vi "Interpolate 2D Scattered_Wn2.vi"(0 "X(Tri) In":dbl[][](array[numeric]), 5 "Y(Tri) In":dbl[][](array[numeric]), 7 "Z(Tri) In":dbl[][](array[numeric]), 9 "gx in":dbl[][](array[numeric]), 11 "gy in":dbl[][](array[numeric]), 12 "Length":dbl[][](array[numeric])) -> (4 "X(Tri) Out":dbl[][](array[numeric]), 6 "Y(Tri) Out":dbl[][](array[numeric]), 8 "Z(Tri) Out":dbl[][](array[numeric]), 10 "gx out":dbl[][](array[numeric]), 14 "Wn 2":dbl[][](array[numeric]), 15 "gy out":dbl[][](array[numeric]))   [LabVIEW 2017, in "NI_AAL_Interpolation.lvlib"]
uses:
  <vilib>/gmath/NI_AAL_Interpolation.lvlib
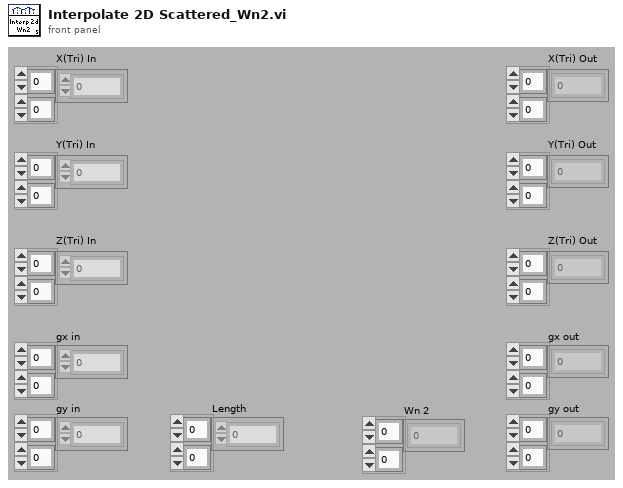
[diagram p1: front panel]
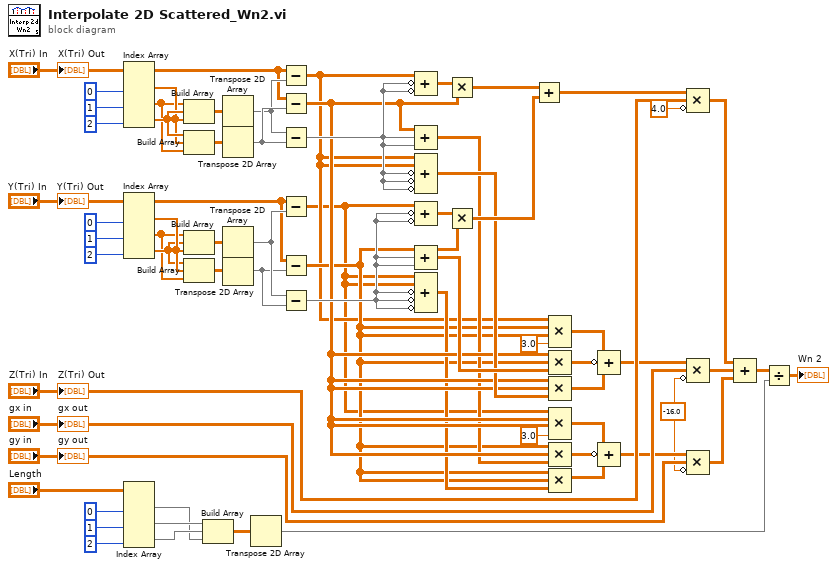
[diagram p0: block diagram]
diagram:
  w8 = -16.0
  n1 = Index Array(array="X(Tri) In", index (col) #1=0 ("disabled index (col)"), index (col) #2=1 ("index (col)"), index (col) #3=2 ("index (col)")) -> (element #1=w59:dbl[], element #2=w58:dbl[], element #3=w60:dbl[])  [unwired: 3 in]
  n2 = Index Array(array="Y(Tri) In", index (col) #1=0 ("disabled index (col)"), index (col) #2=1 ("index (col)"), index (col) #3=2 ("index (col)")) -> (element #1=w57:dbl[], element #2=w55:dbl[], element #3=w56:dbl[])  [unwired: 3 in]
  n3 = Index Array(array="Length", index (col) #1=0 ("disabled index (col)"), index (col) #2=1 ("index (col)"), index (col) #3=2 ("index (col)")) -> (element #1=w40:dbl[], element #2=w42:dbl[], element #3=w41:dbl[])  [unwired: 3 in]
  n4 = Build Array(w58, w60, w59) -> (w52:dbl[][])
  n5 = Build Array(w60, w59, w58) -> (w51:dbl[][])
  n6 = Build Array(w55, w56, w57) -> (w54:dbl[][])
  n7 = Build Array(w56, w57, w55) -> (w53:dbl[][])
  n8 = Build Array(w42, w41, w40) -> (w43:dbl[][])
  n9 = Transpose 2D Array(2D array=w52) -> (transposed array=w44:dbl[][])
  n10 = Transpose 2D Array(2D array=w51) -> (transposed array=w45:dbl[][])
  n11 = Transpose 2D Array(2D array=w54) -> (transposed array=w47:dbl[][])
  n12 = Transpose 2D Array(2D array=w53) -> (transposed array=w46:dbl[][])
  n13 = Transpose 2D Array(2D array=w43) -> (transposed array=w33:dbl[][])
  n14 = Subtract(x="X(Tri) In", y=w44) -> (x-y=w3:dbl[][])
  n15 = Subtract(x="X(Tri) In", y=w45) -> (x-y=w22:dbl[][])
  n16 = Subtract(x=w44, y=w45) -> (x-y=w28:dbl[][])
  n17 = Subtract(x="Y(Tri) In", y=w47) -> (x-y=w2:dbl[][])
  n18 = Subtract(x="Y(Tri) In", y=w46) -> (x-y=w19:dbl[][])
  n19 = Subtract(x=w47, y=w46) -> (x-y=w26:dbl[][])
  n20 = Compound Arithmetic op=ADD(w3, invert w28, invert w28) -> (w32:dbl[][])
  n21 = Compound Arithmetic op=ADD(w22, w28, w28) -> (w21:dbl[][])
  n22 = Compound Arithmetic op=ADD(w3, w3, invert w28, invert w28, invert w28) -> (w24:dbl[][])
  n23 = Compound Arithmetic op=ADD(w2, invert w26, invert w26) -> (w31:dbl[][])
  n24 = Compound Arithmetic op=ADD(w19, w26, w26) -> (w25:dbl[][])
  n25 = Compound Arithmetic op=ADD(w2, w2, invert w26, invert w26, invert w26) -> (w20:dbl[][])
  n26 = Multiply(x=w32, y=w22) -> (x*y=w30:dbl[][])
  n27 = Multiply(x=w31, y=w19) -> (x*y=w29:dbl[][])
  n28 = Add(x=w30, y=w29) -> (x+y=w12:dbl[][])
  n29 = Compound Arithmetic op=MULTIPLY(w3, w19, w19, 3.0) -> (w18:dbl[][])
  n30 = Compound Arithmetic op=MULTIPLY(w22, w19, w25) -> (w17:dbl[][])
  n31 = Compound Arithmetic op=MULTIPLY(w22, w22, w24) -> (w16:dbl[][])
  n32 = Compound Arithmetic op=MULTIPLY(w2, w22, w22, 3.0) -> (w15:dbl[][])
  n33 = Compound Arithmetic op=MULTIPLY(w19, w22, w21) -> (w14:dbl[][])
  n34 = Compound Arithmetic op=MULTIPLY(w19, w19, w20) -> (w13:dbl[][])
  n35 = Compound Arithmetic op=ADD(w18, invert w17, w16) -> (w10:dbl[][])
  n36 = Compound Arithmetic op=ADD(w15, invert w14, w13) -> (w11:dbl[][])
  n37 = Compound Arithmetic op=MULTIPLY(w12, "Z(Tri) In", invert 4.0) -> (w7:dbl[][])
  n38 = Compound Arithmetic op=MULTIPLY(w10, "gx in", invert w8) -> (w6:dbl[][])
  n39 = Compound Arithmetic op=MULTIPLY(w11, "gy in", invert w8) -> (w5:dbl[][])
  n40 = Compound Arithmetic op=ADD(w7, w6, w5) -> (w4:dbl[][])
  n41 = Divide(x=w4, y=w33) -> (x/y=→"Wn 2":dbl[][])
  "X(Tri) Out" <- "X(Tri) In"
  "Y(Tri) Out" <- "Y(Tri) In"
  "Z(Tri) Out" <- "Z(Tri) In"
  "gx out" <- "gx in"
  "gy out" <- "gy in"
